vi "模拟盲打练习键盘(亮灯）.vi"() -> ()   [LabVIEW 2015]
uses:
  <vilib>/Utility/inputDevices.llb/keyboardAcquire.vi
  <vilib>/Utility/inputDevices.llb/closeKeyboard.vi
panel:
  out "Ctrl":bool
  out "BOOKS":bool
  out "*":bool
  out "Alt":bool
  out "Ctrl":bool
  out "*  *\n*  *":bool
  out "?":bool
  out "Alt":bool
  out "|\n\\":bool
  out "Shift":bool
  out "Enter":bool
  out "?\n/":bool
  out ">\n.":bool
  out "\"\n'":bool
  out ":\n;":bool
  out "}\n]":bool
  out "{\n[":bool
  out "Shift":bool
  out "Z":bool
  out "Caps\nLock":bool
  out "<\n ,":bool
  out "M":bool
  out "N":bool
  out "B":bool
  out "V":bool
  out "C":bool
  out "X":bool
  out "Tab":bool
  out "L":bool
  out "K":bool
  out "J":bool
  out "H":bool
  out "G":bool
  out "F":bool
  out "D":bool
  out "S":bool
  out "A":bool
  out "P":bool
  out "O":bool
  out "I":bool
  out "U":bool
  out "Y":bool
  out "T":bool
  out "R":bool
  out "E":bool
  out "W":bool
  out "Q":bool
  in  "停止":bool
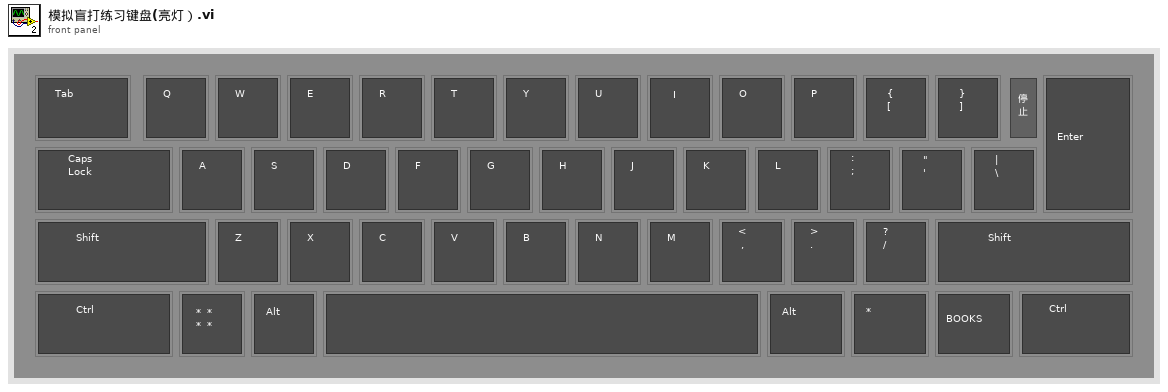
[diagram p1: front panel]
types:
  T1 = enum16{"0", "1", "2", "3", "4", "5", "6", "7", "8", "9", "A", "B", "C", "D", "E", "F", "G", "H", "I", "J", "K", "L", "M", "N", "O", "P", "Q", "R", "S", "T", "U", "V", "W", "X", "Y", "Z", "F1", "F2", "F3", "F4", "F5", "F6", "F7", "F8", "F9", "F10", "F11", "F12", "F13", "F14", "F15", "ADD", "BACK", "BACKSLASH", "CAPITAL", "COMMA", "DECIMAL", "DELETE", "DIVIDE", "DOWN", "END", "EQUALS", "ESCAPE", "GRAVE (`)", "HOME", "INSERT", "LBRACKET", "LCONTROL", "LEFT", "L ALT", "LSHIFT", "LWIN", "MINUS", "MULTIPLY", "NEXT", "NUMLOCK", "NUMPAD_0", "NUMPAD_1", "NUMPAD_2", "NUMPAD_3", "NUMPAD_4", "NUMPAD_5", "NUMPAD_6", "NUMPAD_7", "NUMPAD_8", "NUMPAD_9", "PAUSE", "PERIOD", "PRIOR (PG UP)", "RBRACKET", "RCONTROL", "RETURN", "RIGHT", "R ALT", "RSHIFT", "RWIN", "SCROLL", "SEMICOLON", "SLASH", "SPACE", "SUBTRACT", "TAB", "UP", "ENTER (num pad)", "' (quote)"}
  T2 = enum16{"0", "1", "2", "3", "4", "5", "6", "7", "8", "9", "A", "B", "C", "D", "E", "F", "G", "H", "I", "J", "K", "L", "M", "N", "O", "P", "Q", "R", "S", "T", "U", "V", "W", "X", "Y", "Z", "F1", "F2", "F3", "F4", "F5", "F6", "F7", "F8", "F9", "F10", "F11", "F12", "F13", "F14", "F15", "ADD", "BACK", "BACKSLASH", "CAPITAL", "COMMA", "DECIMAL", "DELETE", "DIVIDE", "DOWN", "END", "EQUALS", "ESCAPE", "GRAVE (`)", "HOME", "INSERT", "LBRACKET", "LCONTROL", "LEFT", "L ALT", "LSHIFT", "LWIN", "MINUS", "MULTIPLY", "NEXT", "NUMLOCK", "NUMPAD_0", "NUMPAD_1", "NUMPAD_2", "NUMPAD_3", "NUMPAD_4", "NUMPAD_5", "NUMPAD_6", "NUMPAD_7", "NUMPAD_8", "NUMPAD_9", "PAUSE", "PERIOD", "PRIOR (PG UP)", "RBRACKET", "RCONTROL", "RETURN", "RIGHT", "R ALT", "RSHIFT", "RWIN", "SCROLL", "SEMICOLON", "SLASH", "SPACE", "SUBTRACT", "TAB", "UP", "ENTER (num pad)", "' (quote)"}[]
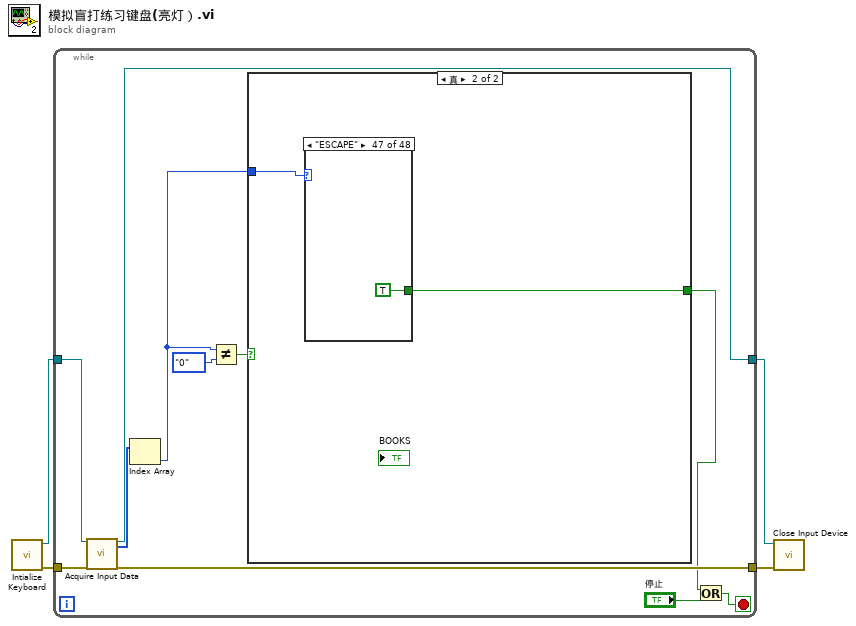
[diagram p0: block diagram]
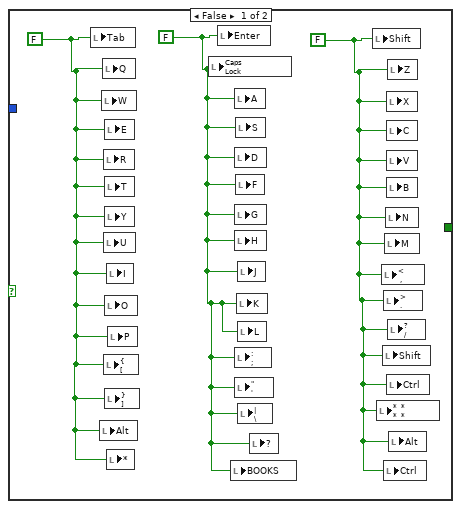
[diagram p2: hidden frame]
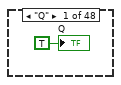
[diagram p3: hidden frame]
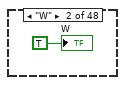
[diagram p4: hidden frame]
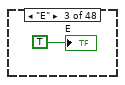
[diagram p5: hidden frame]
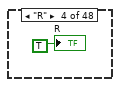
[diagram p6: hidden frame]
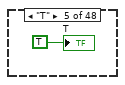
[diagram p7: hidden frame]
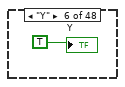
[diagram p8: hidden frame]
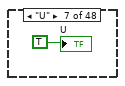
[diagram p9: hidden frame]
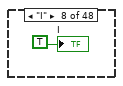
[diagram p10: hidden frame]
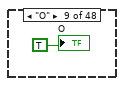
[diagram p11: hidden frame]
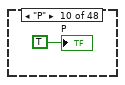
[diagram p12: hidden frame]
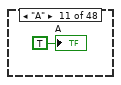
[diagram p13: hidden frame]
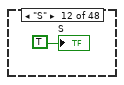
[diagram p14: hidden frame]
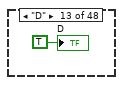
[diagram p15: hidden frame]
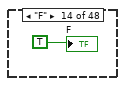
[diagram p16: hidden frame]
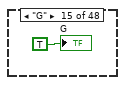
[diagram p17: hidden frame]
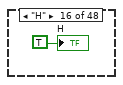
[diagram p18: hidden frame]
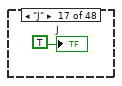
[diagram p19: hidden frame]
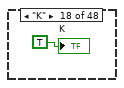
[diagram p20: hidden frame]
diagram:
  n1 = call <vilib>:"Intialize Keyboard.vi"() -> ("error out"=w1:errorcluster, "device ID"=w4:refnum<k1>)  [unwired: 10 in]
  n2 = while {
    tunnel: w4 -> [w15]
    tunnel: [w13] -> w3
    tunnel: [w12] -> w2
    tunnel: w1 -> [w11]
    stop <- w6 stop-if-true
    n3 = call-poly <vilib>:"Acquire Input Data.vi"("device ID"=w15, "error in (no error)"=w11) -> ("device ID"=w12:refnum<k1>, "keys pressed"=w14:T2, "error out"=w13:errorcluster)  [unwired: 15 in]
    n4 = Index Array(array=w14) -> (element=w8:T1)  [unwired: 1 in]
    n5 = Not Equal?(x=w8, y=T1."0") -> (x != y?=w9:bool)
    n6 = case shown="真" w9 {
      tunnel: w8 -> [_ w19]
      tunnel: [_ w20] -> w5
      frame False {
        w16 = FALSE ("x = y?")
        w17 = FALSE ("x = y?")
        w18 = FALSE ("x = y?")
        n7 = local write "Tab"(w18) -> ()
        n8 = local write "Alt"(w18) -> ()
        n9 = local write "W"(w18) -> ()
        n10 = local write "Q"(w18) -> ()
        n11 = local write "R"(w18) -> ()
        n12 = local write "U"(w18) -> ()
        n13 = local write "{\n["(w18) -> ()
        n14 = local write "E"(w18) -> ()
        n15 = local write "T"(w18) -> ()
        n16 = local write "Y"(w18) -> ()
        n17 = local write "O"(w18) -> ()
        n18 = local write "}\n]"(w18) -> ()
        n19 = local write "I"(w18) -> ()
        n20 = local write "*"(w18) -> ()
        n21 = local write "P"(w18) -> ()
        n22 = local write "Caps\nLock"(w17) -> ()
        n23 = local write "Enter"(w17) -> ()
        n24 = local write "BOOKS"(w17) -> ()
        n25 = local write "A"(w17) -> ()
        n26 = local write "D"(w17) -> ()
        n27 = local write "G"(w17) -> ()
        n28 = local write "H"(w17) -> ()
        n29 = local write ":\n;"(w17) -> ()
        n30 = local write "\"\n'"(w17) -> ()
        n31 = local write "S"(w17) -> ()
        n32 = local write "F"(w17) -> ()
        n33 = local write "K"(w17) -> ()
        n34 = local write "J"(w17) -> ()
        n35 = local write "L"(w17) -> ()
        n36 = local write "|\n\\"(w17) -> ()
        n37 = local write item#41(w17) -> ()
        n38 = local write "Shift"(w16) -> ()
        n39 = local write "*  *\n*  *"(w16) -> ()
        n40 = local write "<\n ,"(w16) -> ()
        n41 = local write "Shift"(w16) -> ()
        n42 = local write ">\n."(w16) -> ()
        n43 = local write "Ctrl"(w16) -> ()
        n44 = local write "M"(w16) -> ()
        n45 = local write "N"(w16) -> ()
        n46 = local write "X"(w16) -> ()
        n47 = local write "C"(w16) -> ()
        n48 = local write "V"(w16) -> ()
        n49 = local write "B"(w16) -> ()
        n50 = local write "Ctrl"(w16) -> ()
        n51 = local write "Z"(w16) -> ()
        n52 = local write "?\n/"(w16) -> ()
        n53 = local write "Alt"(w16) -> ()
      }
      frame True {
        n54 = case shown="\"ESCAPE\"" w19 {
          tunnel: [_ _ _ _ _ _ _ _ _ _ _ _ _ _ _ _ _ _ _ _ _ _ _ _ _ _ _ _ _ _ _ _ _ _ _ _ _ _ _ _ _ _ _ _ _ _ TRUE _] -> w20
          frame "Q" {
            "Q" <- TRUE ("Q")
          }
          frame "W" {
            "W" <- TRUE
          }
          frame "E" {
            "E" <- TRUE
          }
          frame "R" {
            "R" <- TRUE
          }
          frame "T" {
            "T" <- TRUE
          }
          frame "Y" {
            "Y" <- TRUE
          }
          frame "U" {
            "U" <- TRUE
          }
          frame "I" {
            "I" <- TRUE
          }
          frame "O" {
            "O" <- TRUE
          }
          frame "P" {
            "P" <- TRUE
          }
          frame "A" {
            "A" <- TRUE
          }
          frame "S" {
            "S" <- TRUE
          }
          frame "D" {
            "D" <- TRUE
          }
          frame "F" {
            "F" <- TRUE
          }
          frame "G" {
            "G" <- TRUE
          }
          frame "H" {
            "H" <- TRUE
          }
          frame "J" {
            "J" <- TRUE
          }
          frame "K" {
            "K" <- TRUE
          }
          frame "L" {
            "L" <- TRUE
          }
          frame "Z" {
            "Z" <- TRUE
          }
          frame "X" {
            "X" <- TRUE
          }
          frame "C" {
            "C" <- TRUE
          }
          frame "V" {
            "V" <- TRUE
          }
          frame "B" {
            "B" <- TRUE
          }
          frame "N" {
            "N" <- TRUE
          }
          frame "M" {
            "M" <- TRUE
          }
          frame "TAB" {
            "Tab" <- TRUE
          }
          frame "CAPITAL" {
            "Caps\nLock" <- TRUE ("Caps\nLock")
          }
          frame "LSHIFT" {
            "Shift" <- TRUE ("Shift")
          }
          frame "LCONTROL" {
            "Ctrl" <- TRUE ("Ctrl")
          }
          frame "LWIN" {
            "*  *\n*  *" <- TRUE ("*  *\n*  *")
          }
          frame "L ALT" {
            "Alt" <- TRUE ("Alt")
          }
          frame "SPACE" {
            "?" <- TRUE
          }
          frame "R ALT" {
            "Alt" <- TRUE ("Alt2")
          }
          frame "RWIN" {
            "*" <- TRUE ("*")
          }
          frame "RCONTROL" {
            "Ctrl" <- TRUE ("* 2")
          }
          frame "LBRACKET" {
            "{\n[" <- TRUE ("* 2")
          }
          frame "RBRACKET" {
            "}\n]" <- TRUE ("}\n]")
          }
          frame "SEMICOLON" {
            ":\n;" <- TRUE (":\n;")
          }
          frame "' (quote)" {
            "\"\n'" <- TRUE ("\"\n'")
          }
          frame "BACKSLASH" {
            "|\n\\" <- TRUE ("|\n\\")
          }
          frame "RETURN" {
            "Enter" <- TRUE ("Enter")
          }
          frame "COMMA" {
            "<\n ," <- TRUE ("<\n ,")
          }
          frame "PERIOD" {
            ">\n." <- TRUE (">\n.")
          }
          frame "SLASH" {
            "?\n/" <- TRUE ("?\n/")
          }
          frame "RSHIFT" {
            "Shift" <- TRUE ("Shift 2")
          }
          frame "ESCAPE" {
          }
          frame Default {
          }
        }
      }
    }
    n55 = Or(x=w5, y="停止") -> (x .or. y?=w6:bool)
  }
  n56 = call-poly <vilib>:"Close Input Device.vi"("error in (no error)"=w3, "device ID"=w2) -> ()  [unwired: 8 in, 1 out]
